vi "Arduino single device test Feb 2017.vi"(5 "# of points to average":i32, 9 "average points?":bool) -> ()   [LabVIEW 2014]
uses:
  <vilib>/Analysis/baseanly.llb/Mean (DBL).vi
  <vilib>/Instr/_visa.llb/VISA Configure Serial Port (Instr).vi
  <vilib>/Analysis/NI_AALBase.lvlib
panel:
  out "Waveform Chart":dbl(graph)
  in  "Stop Button":bool
  in  "Arduino address":refnum<visa-resource-name>
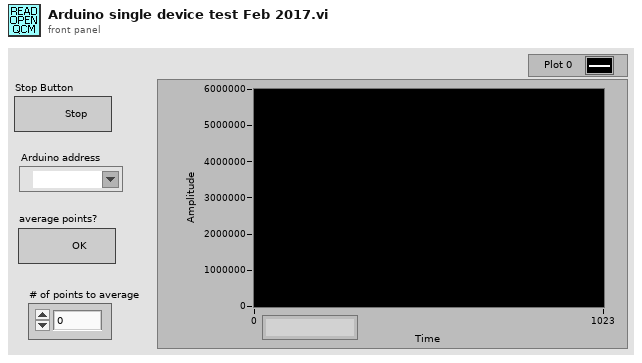
[diagram p1: front panel]
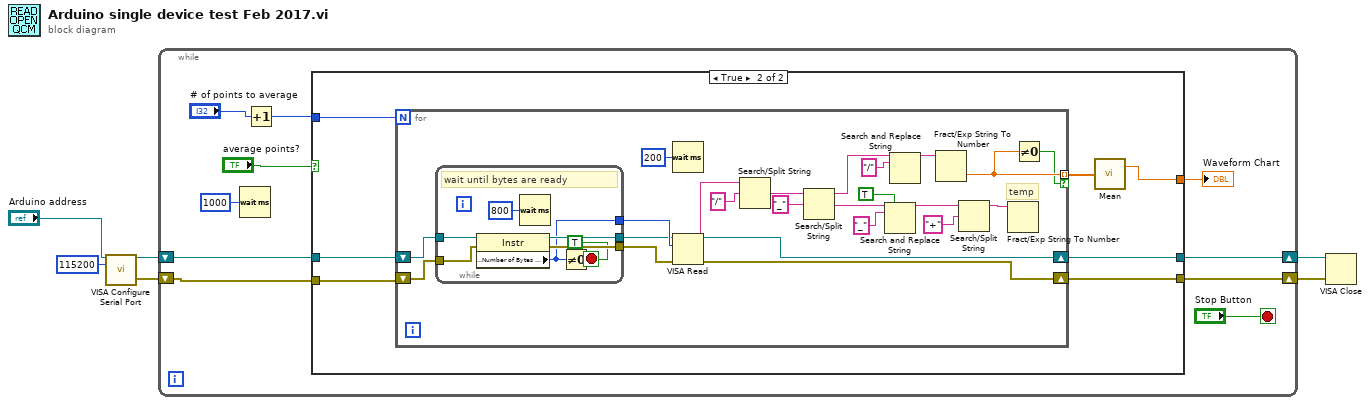
[diagram p0: block diagram]
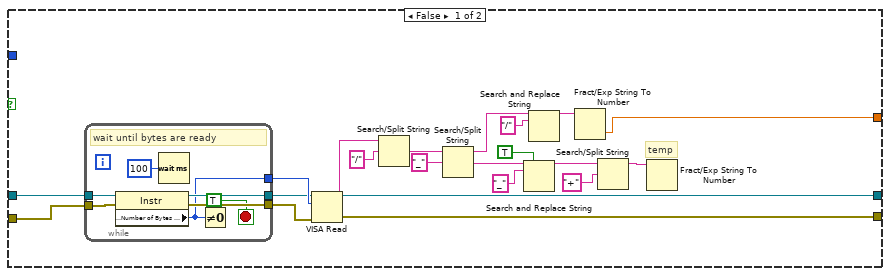
[diagram p2: hidden frame]
diagram:
  n1 = call-poly "VISA Configure Serial Port"("VISA resource name"="Arduino address", "baud rate (9600)"=u32 115200) -> ("VISA resource name out"=w2:refnum<visa-resource-name>, "error out"=w1:errorcluster)  [unwired: 12 in]
  n2 = while {
    shift-right: [w14] -> w4
    shift-left: w2 -> [w11]
    shift-right: [w13] -> w3
    shift-left: w1 -> [w10]
    stop <- "Stop Button" stop-if-true
    n3 = Wait (ms)(milliseconds to wait=u32 1000) -> ()  [unwired: 1 out]
    n4 = Increment(x="# of points to average") -> (x+1=w15:i32)
    n5 = case shown="True" "average points?" {
      tunnel: w11 -> [w21 w51]
      tunnel: w10 -> [w20 w50]
      tunnel: [w18 w49] -> w14
      tunnel: [w19 w48] -> w13
      tunnel: [w17 w45] -> w8
      tunnel: w15 -> [_ w47]
      frame False {
        # "temp"
        n6 = while {
          tunnel: w21 -> [w44]
          tunnel: [w43] -> w23
          tunnel: [w42] -> w22
          tunnel: [w41] -> w24
          tunnel: w20 -> [w38]
          stop <- TRUE stop-if-true
          # "wait until bytes are ready"
          n7 = property class="Instr"(reference=w44, error in=w38) -> (reference out=w42:refnum<visa-resource-name>, error out=w43:errorcluster, "Serial Settings:Number of Bytes at Serial Port"=w41:u32)
          n8 = Wait (ms)(milliseconds to wait=u32 100) -> ()  [unwired: 1 out]
          n9 = Not Equal To 0?(x=w41) -> ()  [unwired: 1 out]
        }
        n10 = VISA Read(VISA resource name=w22, byte count=w24, error in (no error)=w23) -> (VISA resource name out=w18:refnum<visa-resource-name>, read buffer=w37:string, error out=w19:errorcluster)  [unwired: 1 out]
        n11 = Search/Split String(string=w37, search string/char (-)="/") -> (match + rest of string=w30:string)  [unwired: 1 in, 2 out]
        n12 = Search/Split String(string=w30, search string/char (-)="_") -> (substring before match=w36:string, match + rest of string=w31:string)  [unwired: 1 in, 1 out]
        n13 = Search and Replace String(replace all?=TRUE ("replace all? (F)"), input string=w31, search string="_") -> (result string=w25:string)  [unwired: 5 in, 3 out]
        n14 = Search and Replace String(input string=w36, search string="/" ("replace string (\"\")")) -> (result string=w27:string)  [unwired: 6 in, 3 out]
        n15 = Fract/Exp String To Number(string=w27) -> (number=w17:dbl)  [unwired: 3 in, 1 out]
        n16 = Search/Split String(string=w25, search string/char (-)="+") -> (substring before match=w34:string)  [unwired: 1 in, 2 out]
        n17 = Fract/Exp String To Number(string=w34) -> ()  [unwired: 3 in, 2 out]
      }
      frame True {
        n18 = for {
          N: w47 -> [_]
          tunnel: [w53] -> w46 mode=indexing if=w52
          shift-right: [w56] -> w49
          shift-left: w51 -> [w58]
          shift-right: [w55] -> w48
          shift-left: w50 -> [w57]
          # "temp"
          n19 = while {
            tunnel: w57 -> [w80]
            tunnel: w58 -> [w81]
            tunnel: [w79] -> w60
            tunnel: [w78] -> w59
            tunnel: [w77] -> w61
            stop <- TRUE stop-if-true
            # "wait until bytes are ready"
            n20 = property class="Instr"(reference=w81, error in=w80) -> (reference out=w78:refnum<visa-resource-name>, error out=w79:errorcluster, "Serial Settings:Number of Bytes at Serial Port"=w77:u32)
            n21 = Wait (ms)(milliseconds to wait=u32 800) -> ()  [unwired: 1 out]
            n22 = Not Equal To 0?(x=w77) -> ()  [unwired: 1 out]
          }
          n23 = Wait (ms)(milliseconds to wait=u32 200) -> ()  [unwired: 1 out]
          n24 = VISA Read(VISA resource name=w59, byte count=w61, error in (no error)=w60) -> (VISA resource name out=w56:refnum<visa-resource-name>, read buffer=w74:string, error out=w55:errorcluster)  [unwired: 1 out]
          n25 = Search/Split String(string=w74, search string/char (-)="/") -> (match + rest of string=w67:string)  [unwired: 1 in, 2 out]
          n26 = Search/Split String(string=w67, search string/char (-)="_") -> (substring before match=w73:string, match + rest of string=w68:string)  [unwired: 1 in, 1 out]
          n27 = Search and Replace String(replace all?=TRUE ("replace all? (F)"), input string=w68, search string="_") -> (result string=w62:string)  [unwired: 5 in, 3 out]
          n28 = Search and Replace String(input string=w73, search string="/" ("replace string (\"\")")) -> (result string=w64:string)  [unwired: 6 in, 3 out]
          n29 = Fract/Exp String To Number(string=w64) -> (number=w53:dbl)  [unwired: 3 in, 1 out]
          n30 = Search/Split String(string=w62, search string/char (-)="+") -> (substring before match=w71:string)  [unwired: 1 in, 2 out]
          n31 = Fract/Exp String To Number(string=w71) -> ()  [unwired: 3 in, 2 out]
          n32 = Not Equal To 0?(x=w53) -> (x != 0?=w52:bool)
        }
        n33 = call-poly <vilib>:"Mean.vi"("X"=w46) -> ("mean"=w45:dbl)  [unwired: 1 out]
      }
    }
    "Waveform Chart" <- w8
  }
  n34 = VISA Close(VISA resource name=w4, error in (no error)=w3) -> ()  [unwired: 1 out]
